vi "main_6.vi"(0 "Select version":string(combo), 4 "Start":bool, 8 "Stop":bool, 11 "error in (no error)":errorcluster) -> (15 "error out":errorcluster)   [LabVIEW 2023, in "task_6.lvlib"]
doc: "Open the selected labview from the system."
uses:
  task_6.lvlib
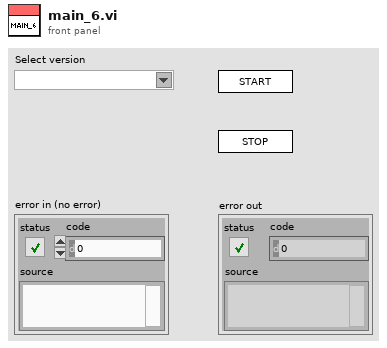
[diagram p1: front panel]
types:
  T1 = typedef "task_6.lvlib/ver_path.ctl" = cluster{"Version":string, "Path":string}
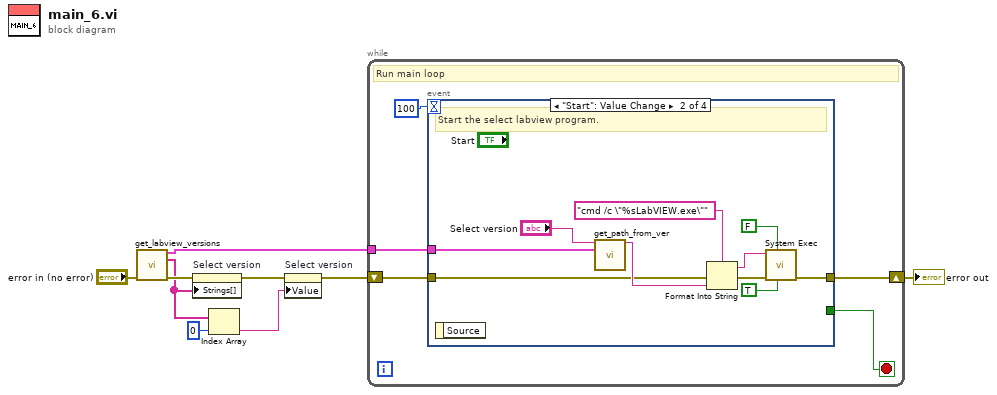
[diagram p0: block diagram]
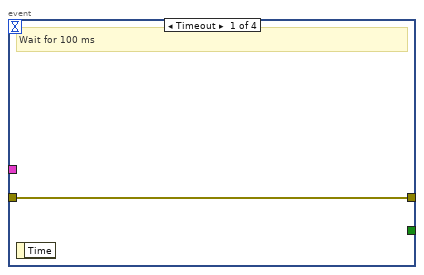
[diagram p2: hidden frame]
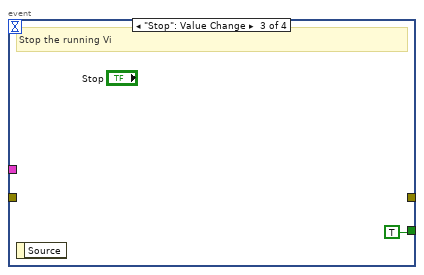
[diagram p3: hidden frame]
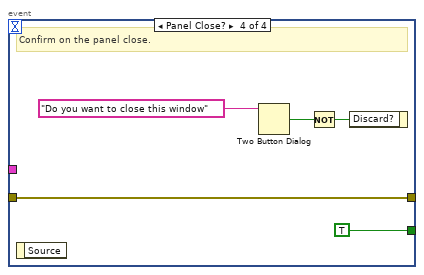
[diagram p4: hidden frame]
diagram:
  n1 = call "get_labview_versions.vi"("error in (no error)"="error in (no error)") -> ("Version with path"=w4:T1[], "Versions"=w3:string[], "error out"=w8:errorcluster)  [unwired: 12 in]
  n2 = property on="Select version" class="CmbBox"(error in=w8, "Strings[]"=w3) -> (error out=w9:errorcluster)  [unwired: 1 in, 1 out]
  n3 = Index Array(array=w3, index=0) -> (element=w5:string)
  n4 = property on="Select version" class="CmbBox"(error in=w9, "Value"=w5) -> (error out=w2:errorcluster)  [unwired: 1 in, 1 out]
  n5 = while {
    tunnel: w4 -> [w12]
    shift-right: [w10] -> w1
    shift-left: w2 -> [w11]
    stop <- w13 stop-if-true
    # "Run main loop"
    n6 = event shown="[1] \"Start\": Value Change" {
      selector: _ -> [_ _ _ _]
      dyn-events: _ -> [_ _ _ _]
      timeout: 100 -> [_ _ _ _]
      tunnel: [_ _ TRUE TRUE] -> w13
      tunnel: w12 -> [_ w25 _ _]
      tunnel: w11 -> [w15 w21 _ w27]
      tunnel: [w15 w16 _ w27] -> w10
      event Timeout {
        # "Wait for 100 ms"
        n7 = event-data() -> ()  [unwired: 1 in, 1 out]
      }
      event "Start": Value Change {
        # "Start the select labview program."
        n8 = event-data() -> ()  [unwired: 1 in, 1 out]
        n9 = call "get_path_from_ver.vi"("Version"="Select version", "Array"=w25) -> ("Path"=w22:string)  [unwired: 13 in]
        n10 = Format Into String(format string="cmd /c \"%sLabVIEW.exe\"", error in=w21, w22) -> (resulting string=w19:string, error out=w20:errorcluster)  [unwired: 1 in]
        n11 = call <vilib>:"System Exec.vi"("run minimized? (F)"=TRUE, "wait until completion? (T)"=FALSE, "error in (no error)"=w20, "command line"=w19) -> ("error out"=w16:errorcluster)  [unwired: 4 in, 3 out]
      }
      event "Stop": Value Change {
        # "Stop the running Vi"
        n12 = event-data() -> ()  [unwired: 1 in, 1 out]
      }
      event Panel Close? {
        # "Confirm on the panel close."
        n13 = event-data() -> ()  [unwired: 1 in, 1 out]
        n14 = Two Button Dialog(message="Do you want to close this window") -> (T button?=w30:bool)  [unwired: 2 in]
        n15 = Not(x=w30) -> (.not. x?=w29:bool)
        n16 = event-data("Discard?"=w29) -> ()  [unwired: 1 in, 1 out]
      }
    }
  }
  "error out" <- w1
